vi "scale-sensors.vi"(0 "Measured Value (mV)":dbl, 1 "Sensor Options":T1) -> (4 "Calculated Value (User Specified Unit)":dbl, 6 "Display Units":string, 10 "Pre Conversion (Sensor True Unit)":dbl, 12 "sensor-range":dbl, 13 "signal-range":dbl, 14 "scaler":dbl)   [LabVIEW 2024]
uses:
  sensor-options.ctl
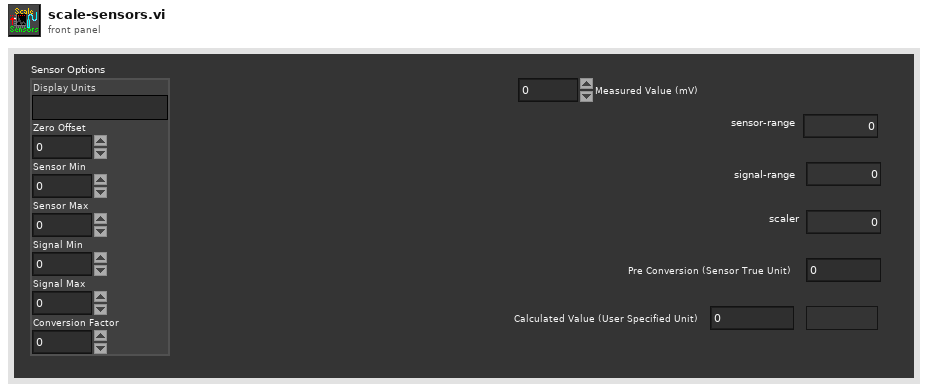
[diagram p1: front panel]
types:
  T1 = typedef "sensor-options.ctl" = cluster{"Display Units":string, "Zero Offset":dbl, "Sensor Min":dbl, "Sensor Max":dbl, "Signal Min":dbl, "Signal Max":dbl, "Conversion Factor":dbl}
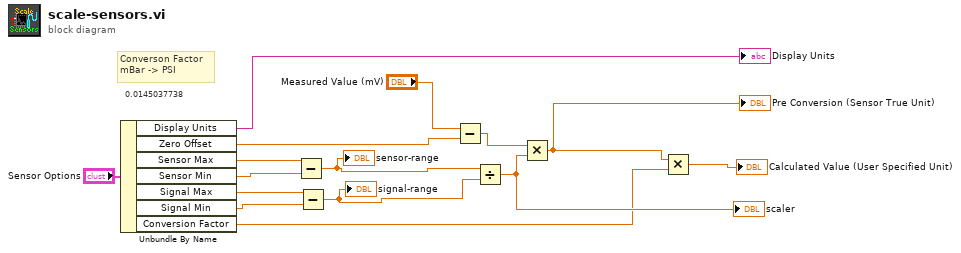
[diagram p0: block diagram]
diagram:
  # "Converson Factor\nmBar -> PSI"
  # "0.0145037738"
  n1 = Unbundle By Name("Sensor Options") -> ("Display Units"=→"Display Units":string, "Zero Offset"=w12:dbl, "Sensor Max"=w11:dbl, "Sensor Min"=w10:dbl, "Signal Max"=w9:dbl, "Signal Min"=w8:dbl, "Conversion Factor"=w3:dbl)
  n2 = Subtract(x=w11, y=w10) -> (x-y=w7:dbl)
  "sensor-range" <- w7
  n3 = Subtract(x=w9, y=w8) -> (x-y=w6:dbl)
  "signal-range" <- w6
  n4 = Subtract(x="Measured Value (mV)", y=w12) -> (x-y=w5:dbl)
  n5 = Divide(x=w7, y=w6) -> (x/y=w4:dbl)
  "scaler" <- w4
  n6 = Multiply(x=w5, y=w4) -> (x*y=w2:dbl)
  "Pre Conversion (Sensor True Unit)" <- w2
  n7 = Multiply(x=w2, y=w3) -> (x*y=→"Calculated Value (User Specified Unit)":dbl)
